vi "Labview_Arduino_Interface.vi"() -> ()   [LabVIEW 2010]
uses:
  <vilib>/Utility/error.llb/DialogType.ctl
  <vilib>/Instr/_visa.llb/VISA Configure Serial Port (Instr).vi
panel:
  in  "x":dbl
  in  "Manual Override":bool
  in  "Valve 3":bool
  in  "Valve 1":bool
  in  "Valve 2":bool
  in  "stop":bool
  in  "baud rate (9600)":u32=9600
  in  "VISA resource name":refnum<visa-resource-name>="COM3"
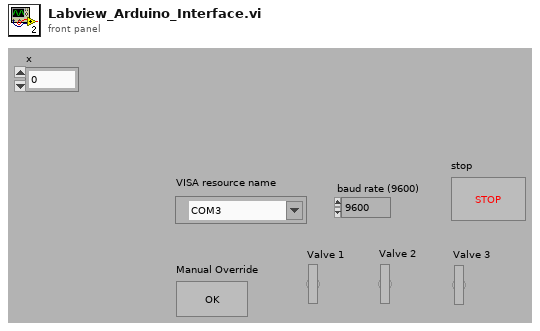
[diagram p1: front panel]
types:
  T1 = typedef "DialogType.ctl" = u16
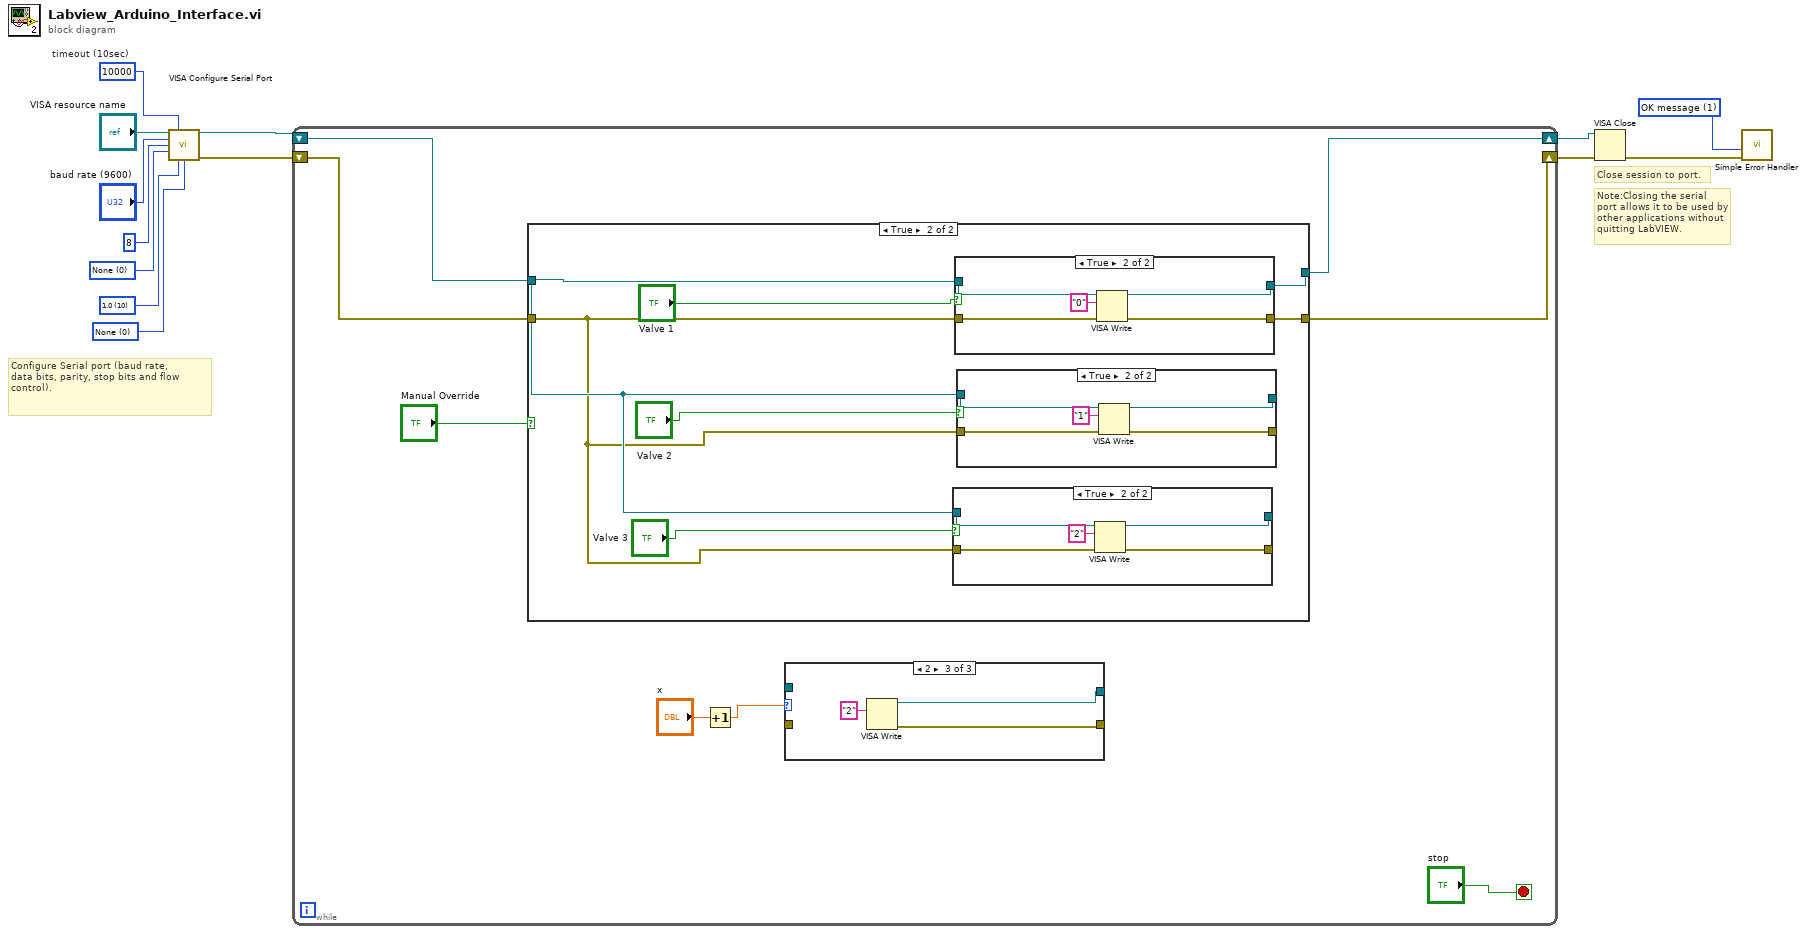
[diagram p0: block diagram]
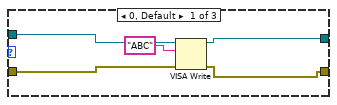
[diagram p2: hidden frame]
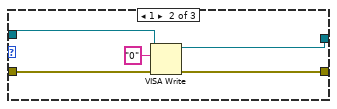
[diagram p3: hidden frame]
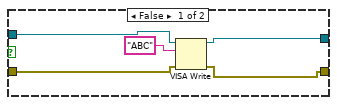
[diagram p5: hidden frame]
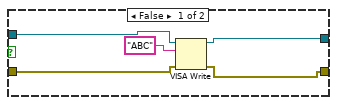
[diagram p6: hidden frame]
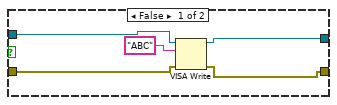
[diagram p7: hidden frame]
diagram:
  w4 = T1 1 items=["no dialog", "OK message", "continue or stop message", "OK message + warnings", "continue/stop + warnings"] ("type of dialog (OK msg:1)")
  w9 = u16 0 items=["None"=0, "XON/XOFF"=1, "RTS/CTS"=2, "DTR/DSR"=4] ("flow control")
  w10 = u16 10 items=["1.0"=10, "1.5"=15, "2.0"=20] ("stop bits")
  w12 = u16 0 items=["None", "Odd", "Even", "Mark", "Space"] ("parity")
  w11 = u32 10000  # timeout (10sec)
  # "Note:Closing the serial port allows it to be used by other applications without\nquitting LabVIEW."
  # "Close session to port."
  # "Configure Serial port (baud rate,\ndata bits, parity, stop bits and flow control)."
  n1 = call-poly "VISA Configure Serial Port"("VISA resource name"="VISA resource name", "timeout (10sec)"=w11, "baud rate (9600)"="baud rate (9600)", "data bits (8)"=u16 8 ("data bits"), "parity (0:none)"=w12, "stop bits (10: 1 bit)"=w10, "flow control (0:none)"=w9) -> ("VISA resource name out"=w1:refnum<visa-resource-name>, "error out"=w2:errorcluster)  [unwired: 2 in, 5 out]
  n2 = while {
    shift-right: [w19] -> w3
    shift-left: w2 -> [w17]
    shift-right: [w20] -> w5
    shift-left: w1 -> [w18]
    stop <- "stop" stop-if-true
    n3 = case shown="True" "Manual Override" {
      tunnel: [w35 w45] -> w20
      tunnel: [w36 w44] -> w19
      tunnel: w18 -> [w38 w40]
      tunnel: w17 -> [w37 w39]
      frame False {
      }
      frame True {
        n4 = case shown="True" "Valve 3" {
          tunnel: [w49 w54] -> _
          tunnel: [w48 w53] -> _
          tunnel: w40 -> [w47 w52]
          tunnel: w39 -> [w46 w51]
          frame False {
            n5 = VISA Write(VISA resource name=w47, write buffer="ABC", error in (no error)=w46) -> (VISA resource name out=w49:refnum<visa-resource-name>, error out=w48:errorcluster)  [unwired: 1 out]
          }
          frame True {
            n6 = VISA Write(VISA resource name=w52, write buffer="2", error in (no error)=w51) -> (VISA resource name out=w54:refnum<visa-resource-name>, error out=w53:errorcluster)  [unwired: 1 out]
          }
        }
        n7 = case shown="True" "Valve 1" {
          tunnel: [w69 w74] -> w45
          tunnel: [w68 w73] -> w44
          tunnel: w40 -> [w67 w72]
          tunnel: w39 -> [w66 w71]
          frame False {
            n8 = VISA Write(VISA resource name=w67, write buffer="ABC", error in (no error)=w66) -> (VISA resource name out=w69:refnum<visa-resource-name>, error out=w68:errorcluster)  [unwired: 1 out]
          }
          frame True {
            n9 = VISA Write(VISA resource name=w72, write buffer="0", error in (no error)=w71) -> (VISA resource name out=w74:refnum<visa-resource-name>, error out=w73:errorcluster)  [unwired: 1 out]
          }
        }
        n10 = case shown="True" "Valve 2" {
          tunnel: [w59 w64] -> _
          tunnel: [w58 w63] -> _
          tunnel: w40 -> [w57 w62]
          tunnel: w39 -> [w56 w61]
          frame False {
            n11 = VISA Write(VISA resource name=w57, write buffer="ABC", error in (no error)=w56) -> (VISA resource name out=w59:refnum<visa-resource-name>, error out=w58:errorcluster)  [unwired: 1 out]
          }
          frame True {
            n12 = VISA Write(VISA resource name=w62, write buffer="1", error in (no error)=w61) -> (VISA resource name out=w64:refnum<visa-resource-name>, error out=w63:errorcluster)  [unwired: 1 out]
          }
        }
      }
    }
    n13 = Increment(x="x") -> (x+1=w15:dbl)
    n14 = case shown="2" w15 {
      tunnel: [w25 w30 w33] -> _
      tunnel: [w24 w29 w32] -> _
      tunnel: _ -> [w23 w28 _]
      tunnel: _ -> [w22 w27 _]
      frame 0, Default {
        n15 = VISA Write(VISA resource name=w23, write buffer="ABC", error in (no error)=w22) -> (VISA resource name out=w25:refnum<visa-resource-name>, error out=w24:errorcluster)  [unwired: 1 out]
      }
      frame 1 {
        n16 = VISA Write(VISA resource name=w28, write buffer="0", error in (no error)=w27) -> (VISA resource name out=w30:refnum<visa-resource-name>, error out=w29:errorcluster)  [unwired: 1 out]
      }
      frame 2 {
        n17 = VISA Write(write buffer="2") -> (VISA resource name out=w33:refnum<visa-resource-name>, error out=w32:errorcluster)  [unwired: 2 in, 1 out]
      }
    }
  }
  n18 = VISA Close(VISA resource name=w5, error in (no error)=w3) -> (error out=w7:errorcluster)
  n19 = call <vilib>:"Simple Error Handler.vi"("type of dialog (OK msg:1)"=w4, "error in (no error)"=w7) -> ()  [unwired: 8 out]
